vi "Test wait continue.vi"() -> ()   [LabVIEW 2018]
panel:
  out "status":T1
  in  "pulse_width_us":dbl=5.0 caption="Pulse width"
  in  "repetitions":i32=10000 caption="Repetitions" min=1 step=1
  in  "sampling_mode":enum16{"Normal", "Sweep"}(ring)=enum."Sweep"
  in  "q_samples":i32=50
  in  "dt_stop_us":dbl=10000.0
  in  "dt_start_us":dbl=0.2
  in  "parameters_recenter":T2={"input_xyz"={"X_um"=0.0, "Y_um"=0.0, "Z_um"=0.0}, "recenter"=FALSE, "recenter_s"=3}
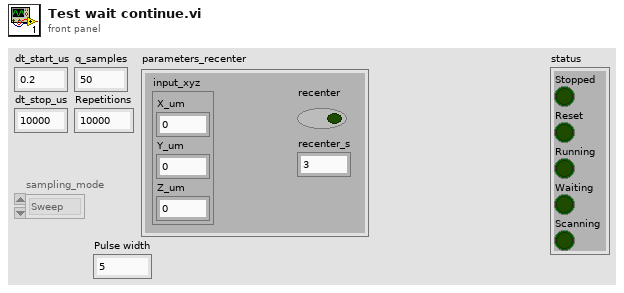
[diagram p1: front panel]
types:
  T1 = cluster{"Stopped":bool, "Reset":bool, "Running":bool, "Waiting":bool, "Scanning":bool}
  T2 = cluster{"input_xyz":cluster{"X_um":sgl, "Y_um":sgl, "Z_um":sgl}, "recenter":bool, "recenter_s":u32}
  T3 = cluster{"MW_width_us":dbl[], "pulse_width_us":dbl, "read_delay_us":dbl, "read_width_us":dbl, "repetitions":i32, "sampling_mode":enum16{"Normal", "Sweep"}, "correction_us":dbl}
  T4 = cluster{"Instruct Data":i32, "Op Code":i32, "Flags":bool[], "Comments":string, "Time":dbl}[]
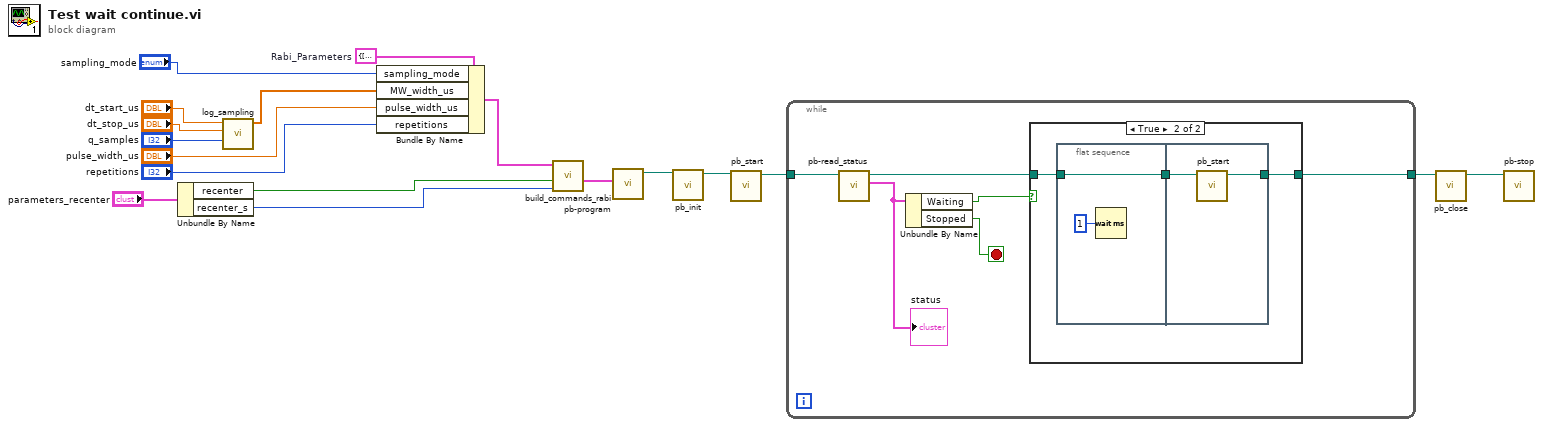
[diagram p0: block diagram]
diagram:
  w14 = T3 {"MW_width_us"=[], "pulse_width_us"=0.0, "read_delay_us"=0.0, "read_width_us"=0.0, "repetitions"=0, "sampling_mode"=enum."Normal", "correction_us"=0.0}  # Rabi_Parameters
  n1 = Unbundle By Name("parameters_recenter") -> ("recenter"=w17:bool, "recenter_s"=w16:u32)
  n2 = call "log_sampling.vi"("q_samples"="q_samples", "stop_us"="dt_stop_us", "start_us"="dt_start_us") -> ("sampling_times_us"=w9:dbl[])  [unwired: 7 in, 1 out]
  n3 = Bundle By Name(cluster=w14, "sampling_mode"="sampling_mode", "MW_width_us"=w9, "pulse_width_us"="pulse_width_us", "repetitions"="repetitions") -> (w6:T3)
  n4 = call "build_commands_rabi.vi"("Refocus_s"=w16, "Refocus?"=w17, "Rabi_parameters"=w6) -> ("commands"=w15:T4)  [unwired: 8 in]
  n5 = call "pb-program.vi"("Commands"=w15) -> ("path out"=w5:path)  [unwired: 10 in]
  n6 = call "pb_init.vi"("path in"=w5) -> ("path out"=w4:path)  [unwired: 9 in, 1 out]
  n7 = call "pb_start.vi"("path in"=w4) -> ("path out"=w3:path)  [unwired: 9 in, 1 out]
  n8 = while {
    tunnel: w3 -> [w21]
    tunnel: [w20] -> w2
    stop <- w19 stop-if-true
    n9 = call "pb-read_status.vi"("path in"=w21) -> ("status"=w24:T1, "path out"=w22:path)  [unwired: 8 in, 1 out]
    "status" <- w24
    n10 = Unbundle By Name(w24) -> ("Waiting"=w23:bool, "Stopped"=w19:bool)
    n11 = case shown="True" w23 {
      tunnel: w22 -> [w25 w28]
      tunnel: [w25 w26] -> w20
      frame False {
      }
      frame True {
        n12 = flat-sequence {
          tunnel: w28 -> [w29]
          tunnel: [w29] -> w27
          tunnel: w27 -> [w32]
          tunnel: [w31] -> w26
          frame #0 {
            n13 = Wait (ms)(milliseconds to wait=u32 1) -> ()  [unwired: 1 out]
          }
          frame #1 {
            n14 = call "pb_start.vi"("path in"=w32) -> ("path out"=w31:path)  [unwired: 9 in, 1 out]
          }
        }
      }
    }
  }
  n15 = call "pb_close.vi"("path in"=w2) -> ("path out"=w1:path)  [unwired: 9 in, 1 out]
  n16 = call "pb-stop.vi"("path in"=w1) -> ()  [unwired: 9 in, 2 out]
